vi "FlatToRichnixnet_grpc_DbGetDBCAttributeRequest.vi"(5 "OutputClusterType":T1, 11 "InputCluster":T3) -> (3 "OutputCluster":T1)   [LabVIEW 2025, in "grpc-xnet_client.lvlib"]
uses:
  nixnet_grpc_DbGetDBCAttributeRequest_Flat.ctl
  nidevice_grpc_Session_Flat.ctl
  nixnet_grpc_GetDBCAttributeMode.ctl
  nixnet_grpc_DbGetDBCAttributeRequest.ctl
  nixnet_grpc_DbGetDBCAttributeRequest_mode_enum/nixnet_grpc_DbGetDBCAttributeRequest_mode_enum.lvclass
  nidevice_grpc_Session.ctl
  grpc-xnet_client.lvlib
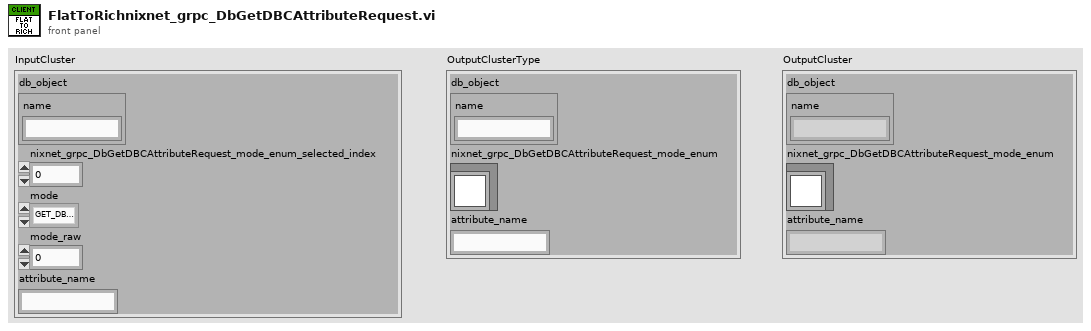
[diagram p1: front panel]
types:
  T1 = typedef "grpc-xnet_client.lvlib/nixnet_grpc_DbGetDBCAttributeRequest.ctl" = cluster{"db_object":T2, "nixnet_grpc_DbGetDBCAttributeRequest_mode_enum":refnum<class "nixnet_grpc_DbGetDBCAttributeRequest_mode_enum.lvclass">, "attribute_name":string}
  T2 = typedef "grpc-xnet_client.lvlib/nidevice_grpc_Session.ctl" = cluster{"name":string}
  T3 = typedef "grpc-xnet_client.lvlib/nixnet_grpc_DbGetDBCAttributeRequest_Flat.ctl" = cluster{"db_object":T4, "nixnet_grpc_DbGetDBCAttributeRequest_mode_enum_selected_index":i32, "mode":T5, "mode_raw":u32, "attribute_name":string}
  T4 = typedef "grpc-xnet_client.lvlib/nidevice_grpc_Session_Flat.ctl" = cluster{"name":string}
  T5 = typedef "grpc-xnet_client.lvlib/nixnet_grpc_GetDBCAttributeMode.ctl" = enum32{"GET_DBC_ATTRIBUTE_MODE_ATTRIBUTE", "GET_DBC_ATTRIBUTE_MODE_ENUMERATION_LIST", "GET_DBC_ATTRIBUTE_MODE_ATTRIBUTE_LIST", "GET_DBC_ATTRIBUTE_MODE_VALUE_TABLE_LIST"}
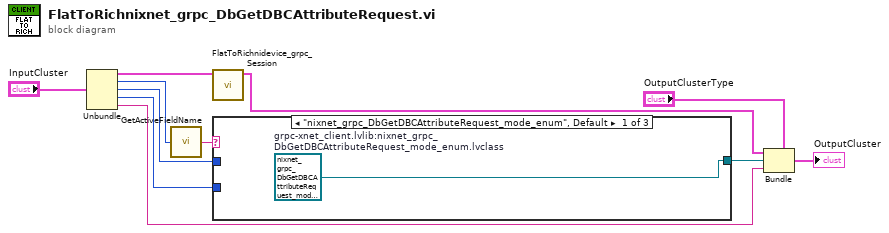
[diagram p0: block diagram]
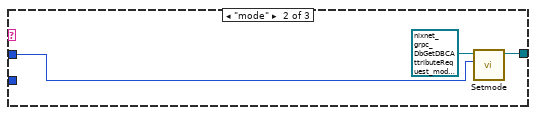
[diagram p2: hidden frame]
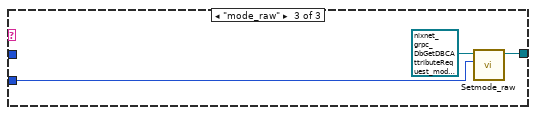
[diagram p3: hidden frame]
diagram:
  n1 = Unbundle "Unbundle"("InputCluster") -> ("db_object"=w8:T4, "nixnet_grpc_DbGetDBCAttributeRequest_mode_enum_selected_index"=w6:i32, "mode"=w3:T5, "mode_raw"=w2:u32, "attribute_name"=w1:string)
  n2 = call "GetActiveFieldName.vi"("protobuf index"=w6) -> ("oneof field name"=w5:string)
  n3 = call "FlatToRichnidevice_grpc_Session.vi"("InputCluster"=w8) -> ("OutputCluster"=w7:T2)  [unwired: 10 in]
  n4 = case "nixnet_grpc_DbGetDBCAttributeRequest_mode_enum" shown="\"nixnet_grpc_DbGetDBCAttributeRequest_mode_enum\", Default" w5 {
    tunnel: [w12 w14 w17] -> w4
    tunnel: w3 -> [_ w15 _]
    tunnel: w2 -> [_ _ w18]
    frame "nixnet_grpc_DbGetDBCAttributeRequest_mode_enum", Default {
      w12 = refnum<class "nixnet_grpc_DbGetDBCAttributeRequest_mode_enum.lvclass"> refnum  # grpc-xnet_client.lvlib:nixnet_grpc_DbGetDBCAttributeRequest_mode_enum.lvclass
    }
    frame "mode" {
      n5 = call "Setmode.vi"("Set_Val"=w15, "OneOfTemplate in"=refnum<class "nixnet_grpc_DbGetDBCAttributeRequest_mode_enum.lvclass"> refnum) -> ("OneOfTemplate out"=w14:refnum<class "nixnet_grpc_DbGetDBCAttributeRequest_mode_enum.lvclass">)  [unwired: 8 in, 1 out]
    }
    frame "mode_raw" {
      n6 = call "Setmode_raw.vi"("Set_Val"=w18, "OneOfTemplate in"=refnum<class "nixnet_grpc_DbGetDBCAttributeRequest_mode_enum.lvclass"> refnum) -> ("OneOfTemplate out"=w17:refnum<class "nixnet_grpc_DbGetDBCAttributeRequest_mode_enum.lvclass">)  [unwired: 8 in, 1 out]
    }
  }
  n7 = Bundle "Bundle"(cluster="OutputClusterType", "db_object"=w7, "nixnet_grpc_DbGetDBCAttributeRequest_mode_enum"=w4, "attribute_name"=w1) -> (→"OutputCluster":T1)
